vi "isALIVE.vi"(8 "error in (no error)":errorcluster, 11 "TecellaClient in":refnum<class "TecellaClient.lvclass">) -> (0 "error out":errorcluster, 2 "Boolean":bool, 3 "TecellaClient out":refnum<class "TecellaClient.lvclass">)   [LabVIEW 2009, in "TecellaClient.lvclass"]
uses:
  TecellaClient.lvclass
panel:
  out "Data Returned":string
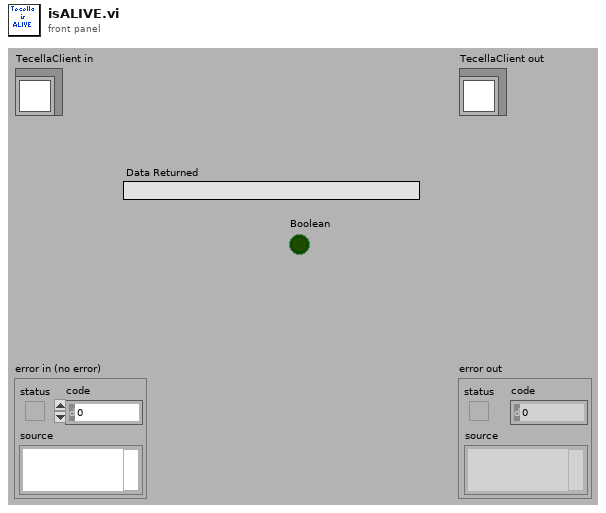
[diagram p1: front panel]
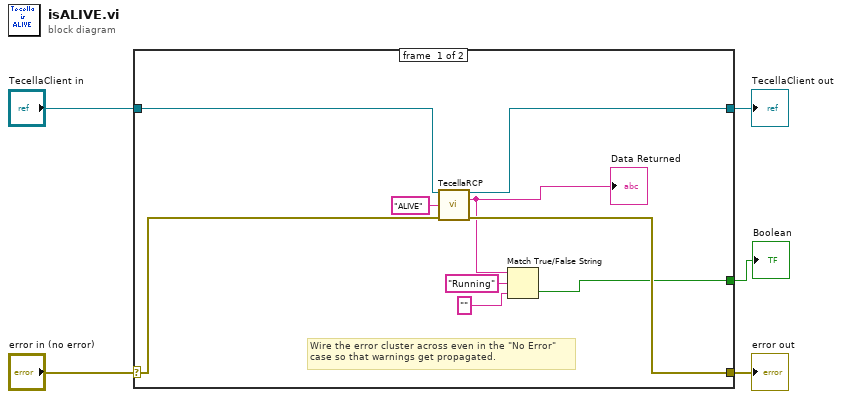
[diagram p0: block diagram]
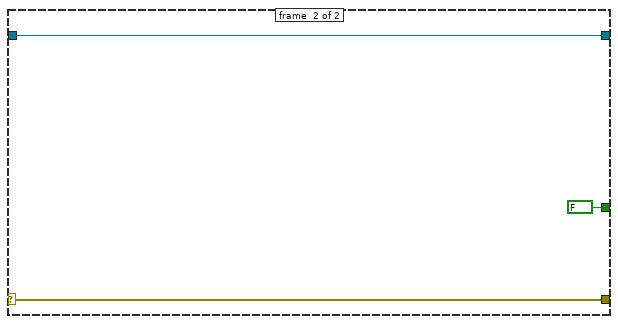
[diagram p2: hidden frame]
diagram:
  n1 = case shown="No Error" "error in (no error)" {
    selector: "error in (no error)" -> [w12 w17]
    tunnel: [w11 w17] -> w4
    tunnel: [w13 w16] -> w2
    tunnel: "TecellaClient in" -> [w14 w16]
    tunnel: [w6 FALSE ("selection")] -> w1
    frame #0 {
      # "Wire the error cluster across even in the \"No Error\"\ncase so that warnings get propagated."
      n2 = call-dynamic "TecellaRCP.vi"("TecellaClient in"=w14, "method"="ALIVE", "error in (no error)"=w12) -> ("TecellaClient out"=w13:refnum<class "TecellaClient.lvclass">, "Data Returned"=w9:string, "error out"=w11:errorcluster)  [unwired: 10 in]
      "Data Returned" <- w9
      n3 = Match True/False String(2:"" ("false string"), 3:"Running" ("true string"), 4:w9) -> (0:w6:bool)  [unwired: 1 out]
    }
    frame #1 {
    }
  }
  "error out" <- w4
  "TecellaClient out" <- w2
  "Boolean" <- w1
